vi "fitting_1d_pixel.vi"(6 "D sign":dbl, 7 "side velocity threshold":dbl, 8 "fitting axis":dbl, 9 "ratio_pixel2mil":dbl, 11 "array in":dbl[][](array[numeric])) -> (0 "D":ext[](array[numeric]), 3 "fitting array":dbl[][](array[numeric]))   [LabVIEW 2017]
uses:
  <vilib>/Analysis/NI_AALPro.lvlib
panel:
  out "Array out 2":ext[](array[numeric])
  out "Array out":ext[](array[numeric])
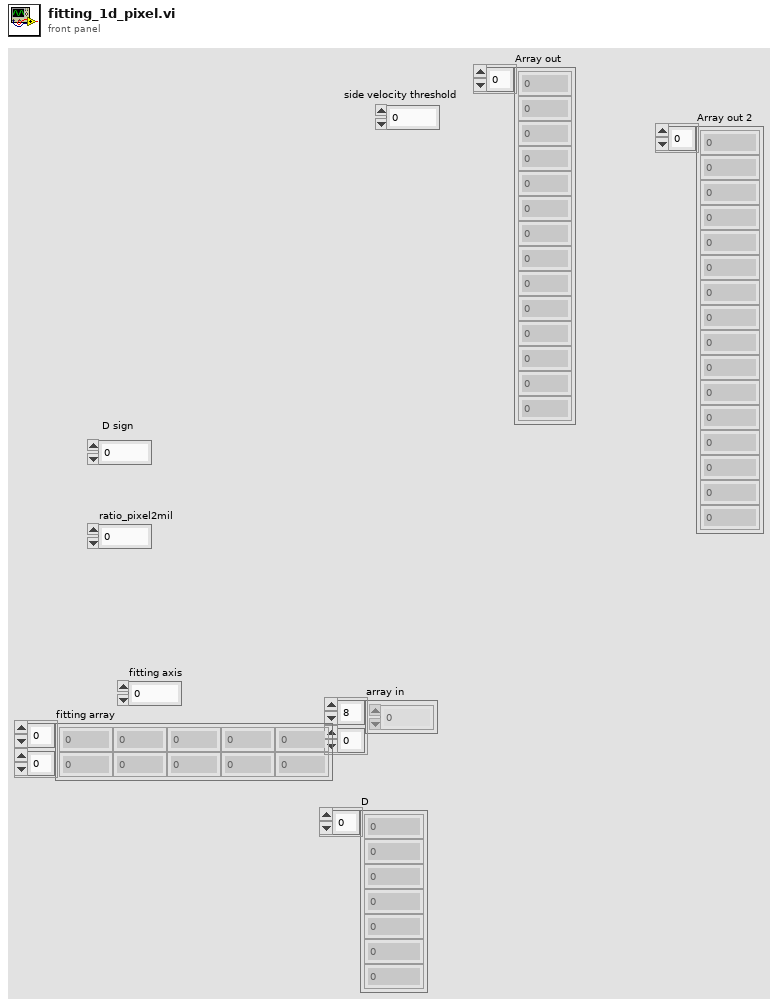
[diagram p1: front panel]
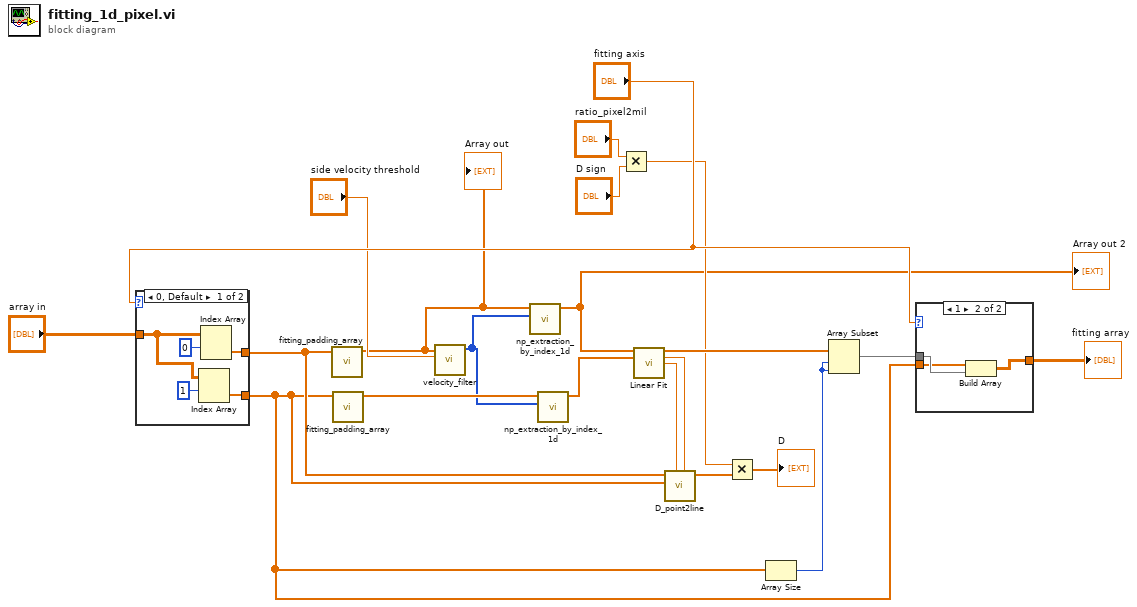
[diagram p0: block diagram]
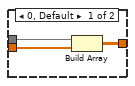
[diagram p2: hidden frame]
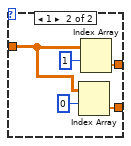
[diagram p3: hidden frame]
diagram:
  n1 = case shown="0, Default" "fitting axis" {
    tunnel: "array in" -> [w24 w29]
    tunnel: [w23 w28] -> w15
    tunnel: [w22 w27] -> w14
    frame 0, Default {
      n2 = Index Array(array=w24, index (row)=1) -> (element=w22:dbl[])  [unwired: 1 in]
      n3 = Index Array(array=w24, index (row)=0) -> (element=w23:dbl[])  [unwired: 1 in]
    }
    frame 1 {
      n4 = Index Array(array=w29, index (row)=0) -> (element=w27:dbl[])  [unwired: 1 in]
      n5 = Index Array(array=w29, index (row)=1) -> (element=w28:dbl[])  [unwired: 1 in]
    }
  }
  n6 = call "fitting_padding_array.vi"("array in"=w15) -> ("Array out"=w1:ext[])  [unwired: 10 in]
  "Array out" <- w1
  n7 = call "fitting_padding_array.vi"("array in"=w14) -> ("Array out"=w5:ext[])  [unwired: 10 in]
  n8 = call "velocity_filter.vi"("threshold"="side velocity threshold", "Array in"=w1) -> ("index"=w4:i32[])  [unwired: 9 in]
  n9 = call "np_extraction_by_index_1d.vi"("index array"=w4, "Array in"=w1) -> ("Array out"=w2:ext[])  [unwired: 9 in]
  "Array out 2" <- w2
  n10 = call "np_extraction_by_index_1d.vi"("index array"=w4, "Array in"=w5) -> ("Array out"=w3:ext[])  [unwired: 9 in]
  n11 = Multiply(x="ratio_pixel2mil", y="D sign") -> (x*y=w7:dbl)
  n12 = call <vilib>:"Linear Fit.vi"("Y"=w2, "X"=w3) -> ("Best Linear Fit"=w20:dbl[], "slope"=w17:dbl, "intercept"=w16:dbl)  [unwired: 9 in, 2 out]
  n13 = call "D_point2line.vi"("slope"=w17, "intercept"=w16, "X Array"=w14, "Y Array"=w15) -> ("D"=w12:ext[])  [unwired: 5 in, 2 out]
  n14 = Multiply(x=w7, y=w12) -> (x*y=→"D":ext[])
  n15 = Array Size(array=w14) -> (size(s)=w21:i32)
  n16 = Array Subset(array=w20, index=w21, length=w21) -> (w19:dbl[])
  n17 = case shown="1" "fitting axis" {
    tunnel: w19 -> [w34 w36]
    tunnel: w14 -> [w33 w35]
    tunnel: [w32 w37] -> w11
    frame 0, Default {
      n18 = Build Array(w34, w33) -> (w32:dbl[][])
    }
    frame 1 {
      n19 = Build Array(w35, w36) -> (w37:dbl[][])
    }
  }
  "fitting array" <- w11
